vi "AvgStd.vi"(8 "error in (no error)":errorcluster, 10 "Tolerance":dbl=0.001 min=0.001, 11 "Value in":dbl[](array[numeric])) -> (0 "error out":errorcluster, 2 "Mean value":dbl)   [LabVIEW 2020]
uses:
  <vilib>/Analysis/baseanly.llb/Mean (DBL).vi
  <vilib>/Analysis/NI_AALBase.lvlib
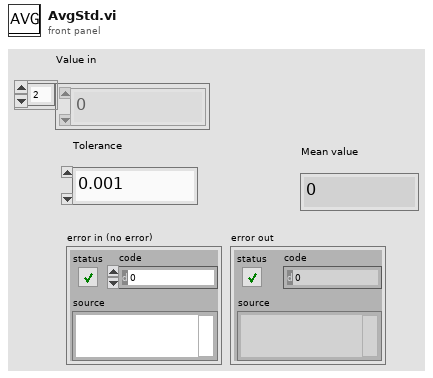
[diagram p1: front panel]
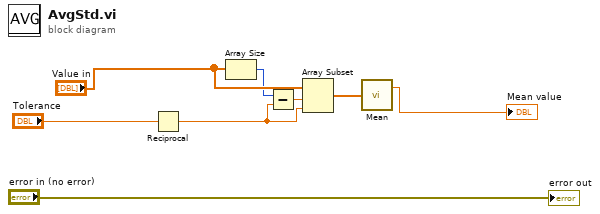
[diagram p0: block diagram]
diagram:
  n1 = Reciprocal(x="Tolerance") -> (1/x=w2:dbl)
  n2 = Array Size(array="Value in") -> (size(s)=w3:i32)
  n3 = Subtract(x=w3, y=w2) -> (x-y=w1:dbl)
  n4 = Array Subset(array="Value in", index=w1, length=w2) -> (w8:dbl[])
  n5 = call-poly <vilib>:"Mean.vi"("X"=w8) -> ("mean"=→"Mean value":dbl)  [unwired: 1 out]
  "error out" <- "error in (no error)"
